vi "Find Quadrant.vi"(11 "Image Coordinate":refnum<class "Vec3d Class.lvclass">) -> (3 "Quadrant":i32)   [LabVIEW 2011]
uses:
  Vec3d Class/Vec3d Class.lvclass
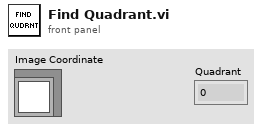
[diagram p1: front panel]
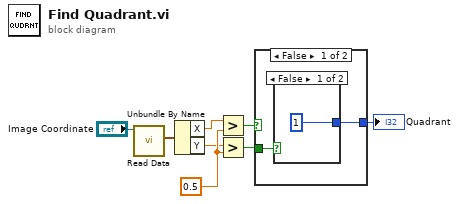
[diagram p0: block diagram]
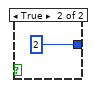
[diagram p2: hidden frame]
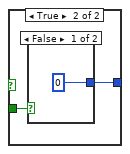
[diagram p3: hidden frame]
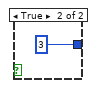
[diagram p4: hidden frame]
diagram:
  w5 = 0.5
  n1 = call-dynamic "Read Data.vi"("Vec3d Class in"="Image Coordinate") -> ("Data"=w7:cluster{"X":dbl, "Y":dbl, "Z":dbl})  [unwired: 8 in, 2 out]
  n2 = Unbundle By Name(w7) -> ("X"=w4:dbl, "Y"=w3:dbl)
  n3 = Greater?(x=w4, y=w5) -> (0:w1:bool)
  n4 = Greater?(x=w3, y=w5) -> (0:w2:bool)
  n5 = case shown="False" w1 {
    tunnel: w2 -> [w10 w14]
    tunnel: [w9 w13] -> w6
    frame False {
      n6 = case shown="False" w10 {
        tunnel: [1 2] -> w9
        frame False {
        }
        frame True {
        }
      }
    }
    frame True {
      n7 = case shown="False" w14 {
        tunnel: [0 3] -> w13
        frame False {
        }
        frame True {
        }
      }
    }
  }
  "Quadrant" <- w6
